vi "CLD 12 Sequencer State Machine.vi"() -> ()   [LabVIEW 2014]
doc: "CLD-Übung 12"
uses:
  CLD 12 Sequencer Enum.ctl
  CLD12 Timer Enum.ctl
  CLD 12 Data Cluster.ctl
panel:
  out "Aktuelle Zielzeit":dbl
  in  "Stopp-Schaltfläche":bool
  out "Verstrichene Zeit":dbl
  out "Schalter 3":bool
  out "Schalter 2":bool
  out "Schalter 1":bool
  in  "Start":bool
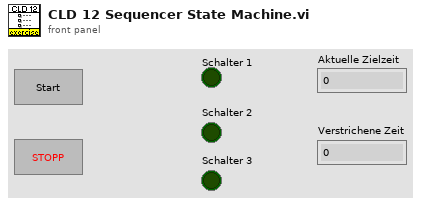
[diagram p1: front panel]
types:
  T1 = typedef "CLD 12 Sequencer Enum.ctl" = enum16{"Initialisieren", "SetTime", "RunState1", "Runstate2", "Ruhezustand", "Starten"}
  T2 = typedef "CLD12 Timer Enum.ctl" = enum16{"Timer starten", "Zeit lesen", "Anhalten", "Fortsetzen", "Timer zurücksetzen"}
  T3 = typedef "CLD 12 Data Cluster.ctl" = cluster{"Befehl":T1, "Zeitwert":dbl, "Boolesch":bool, "Boolesch 2":bool, "Boolesch 3":bool}
  T4 = cluster{"Status":bool, "Code":i32, "Quelle":string}
  T5 = cluster{string, "Zeitwert":dbl, "Boolesch":bool, "Boolesch 2":bool, "Boolesch 3":bool}
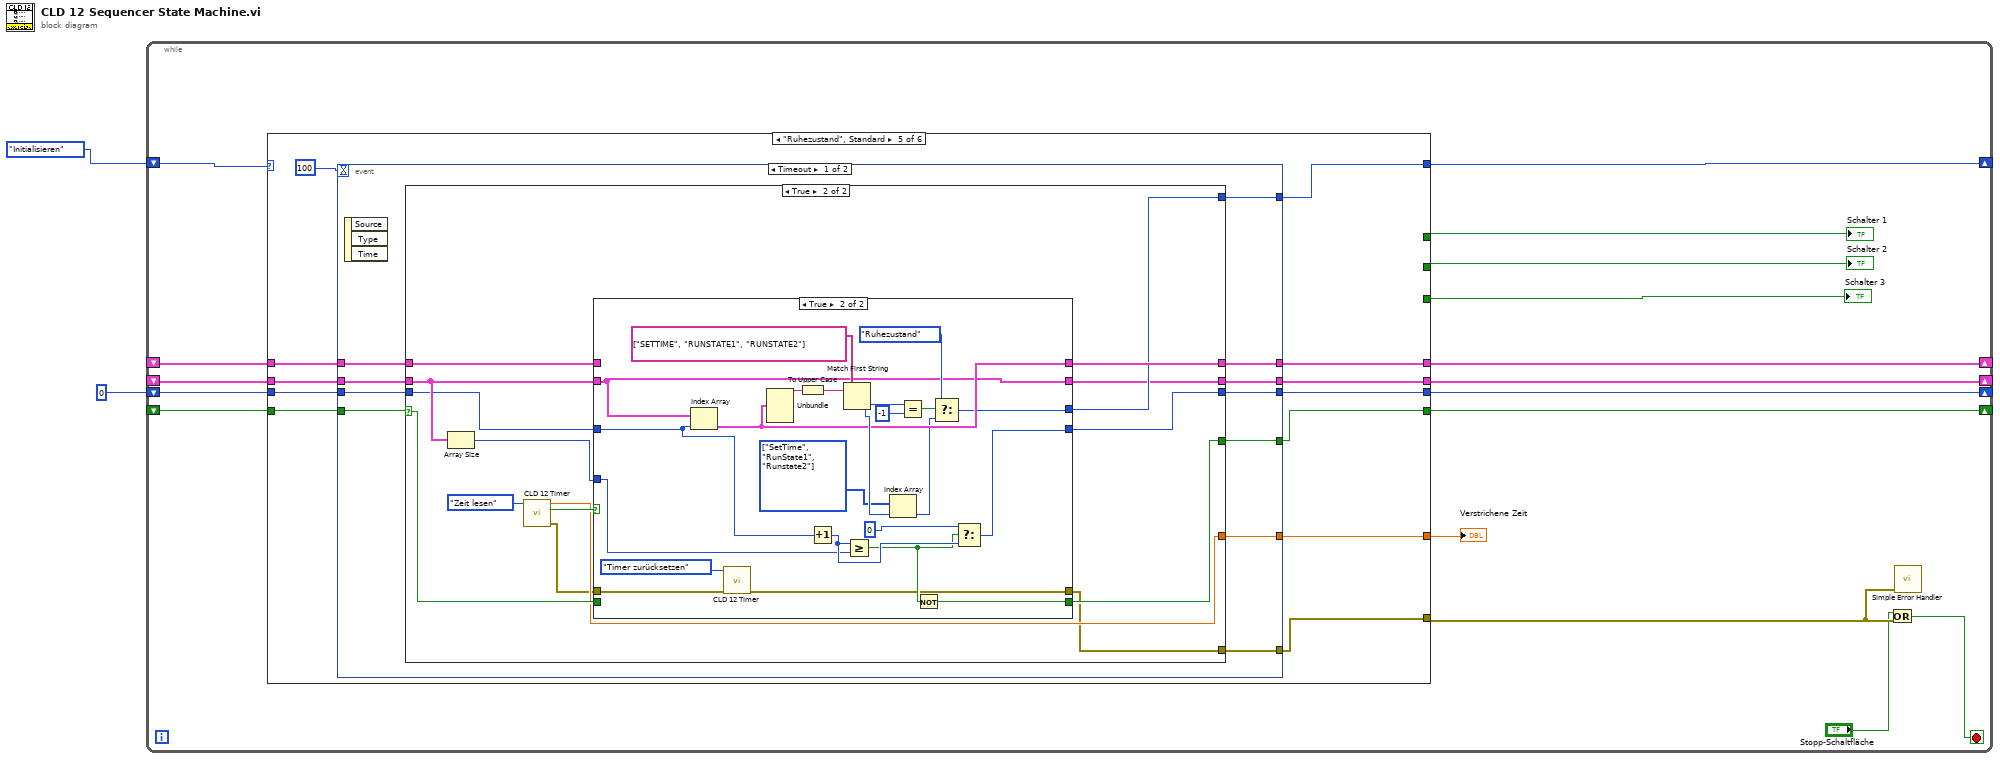
[diagram p0: block diagram]
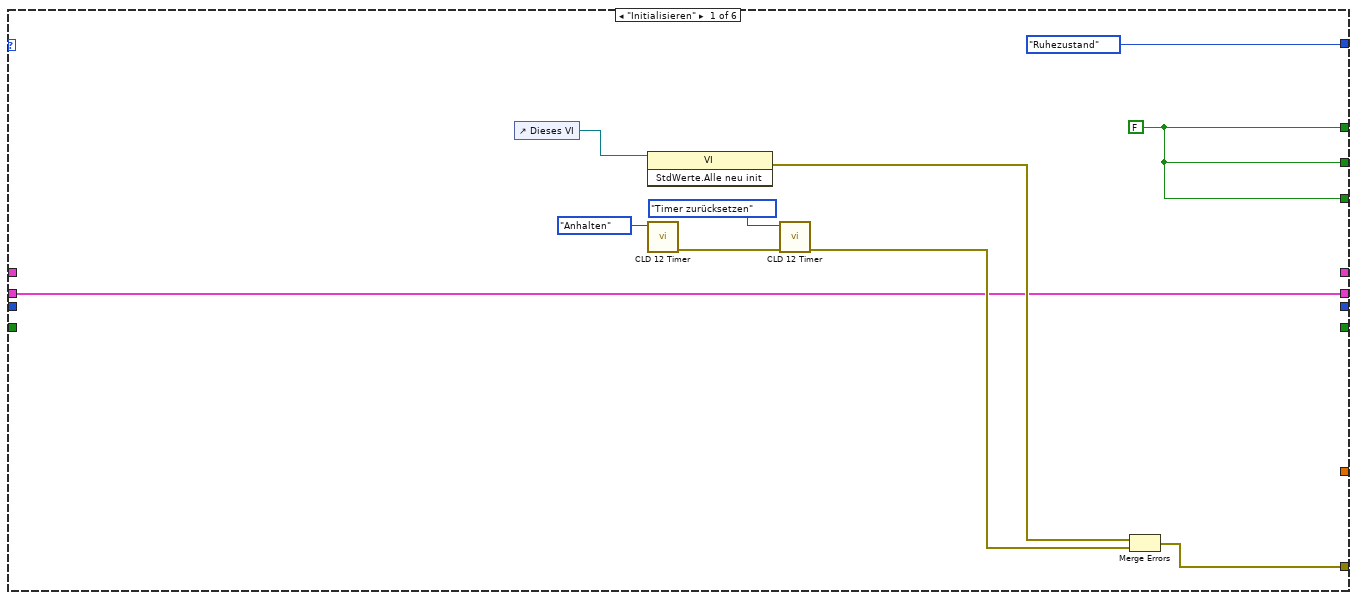
[diagram p2: hidden frame]
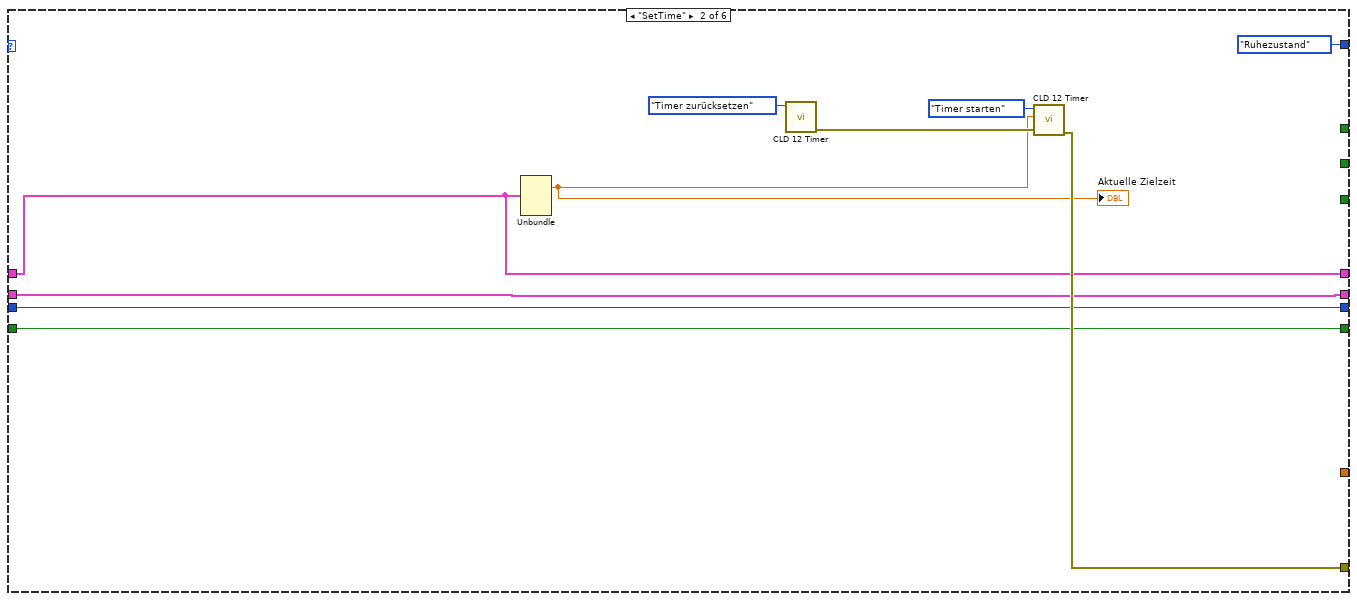
[diagram p3: hidden frame]
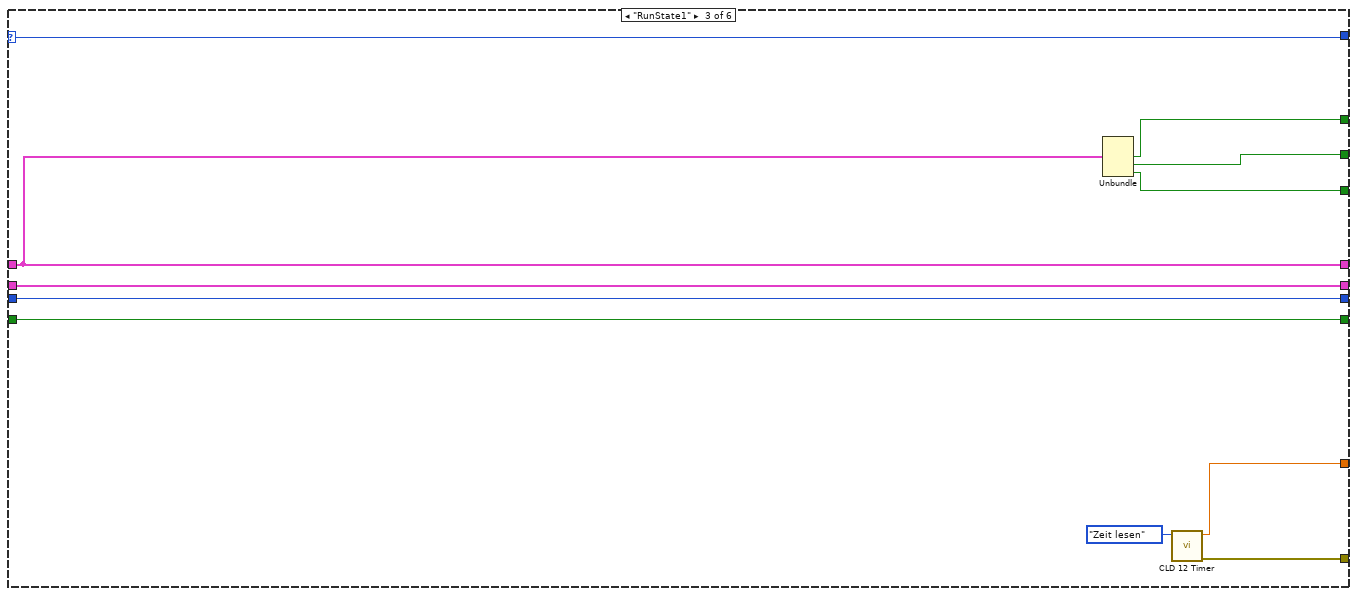
[diagram p4: hidden frame]
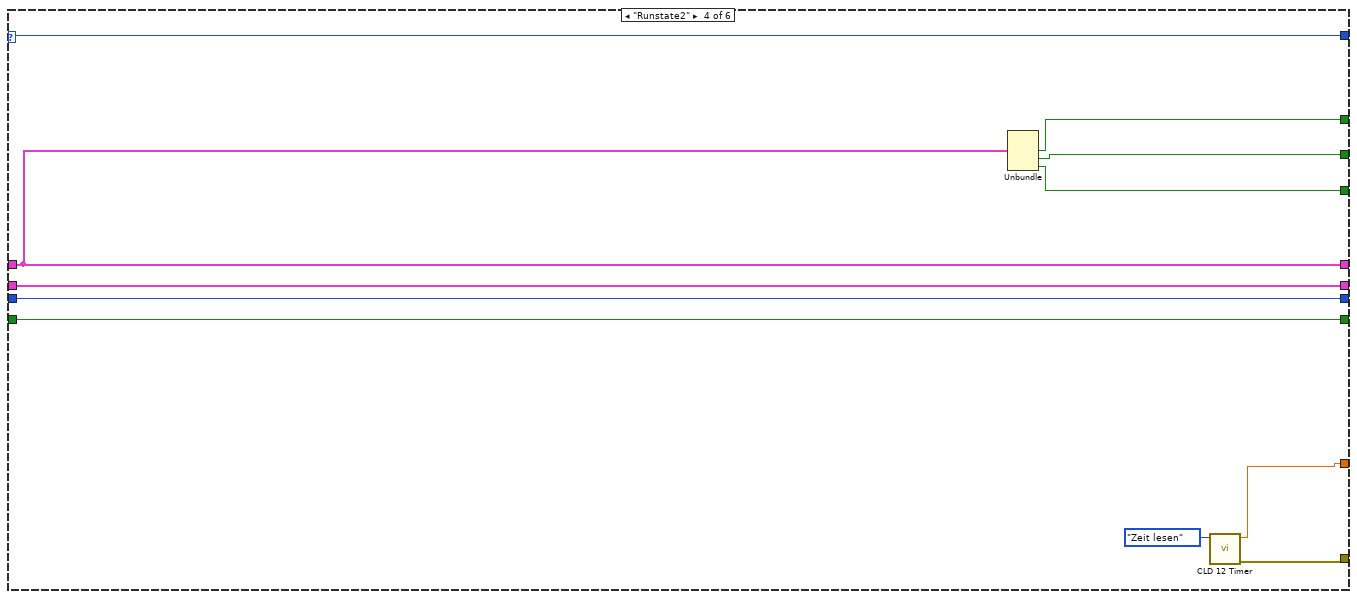
[diagram p5: hidden frame]
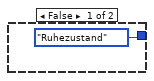
[diagram p6: hidden frame]
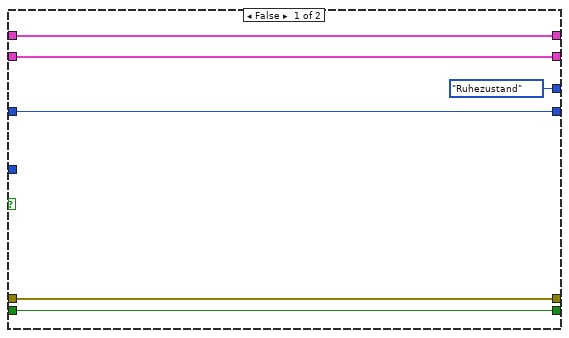
[diagram p7: hidden frame]
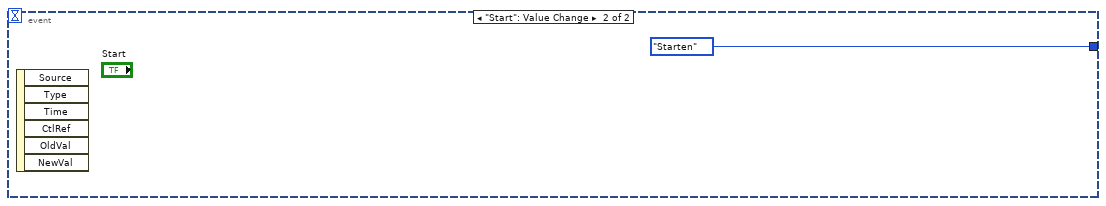
[diagram p8: hidden frame]
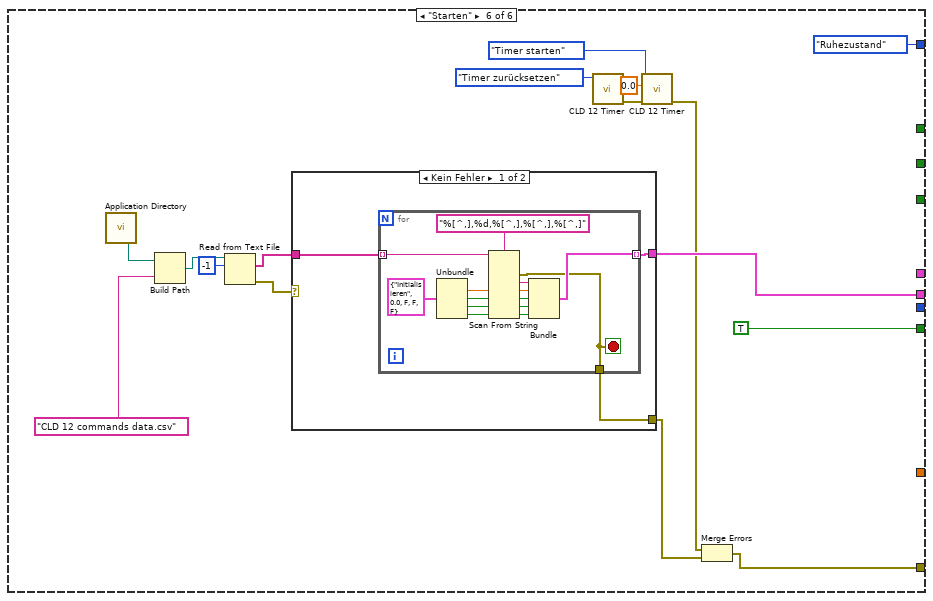
[diagram p9: hidden frame]
diagram:
  n1 = while {
    shift-right: [w10] -> _
    shift-left: CLD_12_Sequencer_Enum."Initialisieren" ("CLD 12 - Sequenzierelement") -> [w9]
    shift-right: [w14] -> _
    shift-left: _ -> [w8]
    shift-right: [w12] -> _
    shift-left: 0 -> [w5]
    shift-right: [w13] -> _
    shift-left: _ -> [w4]
    shift-right: [w6] -> _
    shift-left: _ -> [w7]
    stop <- w16 stop-if-true
    n2 = case shown="\"Ruhezustand\", Standard" w9 {
      selector: w9 -> [_ _ w50 w61 _ _]
      tunnel: [w28 _ w49 w60 _ _] -> w19
      tunnel: [w28 _ w48 w59 _ _] -> w18
      tunnel: [w28 _ w47 w58 _ _] -> w17
      tunnel: [w24 w38 w46 w56 w63 w136] -> w15
      tunnel: [w20 w34 w42 w54 w66 w137] -> w14
      tunnel: [_ w32 w40 w53 w65 TRUE] -> w13
      tunnel: [CLD_12_Sequencer_Enum."Ruhezustand" ("CLD 12 - Sequenzierelement") CLD_12_Sequencer_Enum."Ruhezustand" ("Befehl") w50 w61 w72 CLD_12_Sequencer_Enum."Ruhezustand" ("Befehl")] -> w10
      tunnel: [_ w33 w43 w51 w67 _] -> w12
      tunnel: w8 -> [w20 w34 w42 w54 w71 _]
      tunnel: w7 -> [_ w31 w41 w52 w69 _]
      tunnel: [_ w31 w41 w52 w70 _] -> w6
      tunnel: w5 -> [_ w33 w43 w51 w68 _]
      tunnel: w4 -> [_ w32 w40 w53 w64 _]
      tunnel: [_ _ w45 w55 w62 _] -> w3
      frame "Initialisieren" {
        w28 = FALSE
        n3 = control-ref of="Dieses VI"() -> (w29:refnum<vi>)
        n4 = invoke class="VI" method="StdWerte.Alle neu init"(reference=w29) -> (error out=w26:errorcluster)  [unwired: 2 in, 2 out]
        n5 = call "CLD 12 Timer.vi"("CLD 12 - Timer-Enum"=CLD12_Timer_Enum."Anhalten") -> ("Fehler (Ausgang)"=w25:T4)  [unwired: 8 in, 2 out]
        n6 = call "CLD 12 Timer.vi"("Fehler (Eingang)"=w25, "CLD 12 - Timer-Enum"=CLD12_Timer_Enum."Timer zurücksetzen") -> ("Fehler (Ausgang)"=w23:T4)  [unwired: 7 in, 2 out]
        n7 = Merge Errors(w26, w23) -> (w24:errorcluster)
      }
      frame "SetTime" {
        n8 = Unbundle(w31) -> ("Zeitwert"=w35:dbl)  [unwired: 4 out]
        "Aktuelle Zielzeit" <- w35
        n9 = call "CLD 12 Timer.vi"("CLD 12 - Timer-Enum"=CLD12_Timer_Enum."Timer zurücksetzen") -> ("Fehler (Ausgang)"=w37:T4)  [unwired: 8 in, 2 out]
        n10 = call "CLD 12 Timer.vi"("Fehler (Eingang)"=w37, "Zielzeit (s)"=w35, "CLD 12 - Timer-Enum"=CLD12_Timer_Enum."Timer starten") -> ("Fehler (Ausgang)"=w38:T4)  [unwired: 6 in, 2 out]
      }
      frame "RunState1" {
        n11 = Unbundle(w41) -> ("Boolesch"=w49:bool, "Boolesch 2"=w48:bool, "Boolesch 3"=w47:bool)  [unwired: 2 out]
        n12 = call "CLD 12 Timer.vi"("CLD 12 - Timer-Enum"=CLD12_Timer_Enum."Zeit lesen") -> ("Fehler (Ausgang)"=w46:T4, "Verstrichene Zeit (s,ms)"=w45:dbl)  [unwired: 8 in, 1 out]
      }
      frame "Runstate2" {
        n13 = Unbundle(w52) -> ("Boolesch"=w60:bool, "Boolesch 2"=w59:bool, "Boolesch 3"=w58:bool)  [unwired: 2 out]
        n14 = call "CLD 12 Timer.vi"("CLD 12 - Timer-Enum"=CLD12_Timer_Enum."Zeit lesen") -> ("Fehler (Ausgang)"=w56:T4, "Verstrichene Zeit (s,ms)"=w55:dbl)  [unwired: 8 in, 1 out]
      }
      frame "Ruhezustand", Default {
        n15 = event shown="[0] Timeout" {
          selector: _ -> [_ _]
          dyn-events: _ -> [_ _]
          timeout: 100 -> [_ _]
          tunnel: [w84 _] -> w70
          tunnel: [w83 CLD_12_Sequencer_Enum."Starten" ("Befehl")] -> w72
          tunnel: [w82 _] -> w67
          tunnel: [w80 _] -> w65
          tunnel: [w81 _] -> w63
          tunnel: w71 -> [w79 _]
          tunnel: w69 -> [w78 _]
          tunnel: w68 -> [w77 _]
          tunnel: [w76 _] -> w66
          tunnel: w64 -> [w75 _]
          tunnel: [w74 _] -> w62
          event Timeout {
            n16 = event-data() -> ()  [unwired: 1 in, 3 out]
            n17 = case shown="True" w75 {
              selector: w75 -> [_ w96]
              tunnel: [_ w94] -> w84
              tunnel: [CLD_12_Sequencer_Enum."Ruhezustand" ("Befehl") w93] -> w83
              tunnel: [_ w97] -> w82
              tunnel: [_ w86] -> w81
              tunnel: [_ w95] -> w80
              tunnel: w79 -> [_ w91]
              tunnel: w78 -> [_ w92]
              tunnel: w77 -> [_ w90]
              tunnel: [_ w89] -> w76
              tunnel: [_ w88] -> w74
              frame False {
              }
              frame True {
                n18 = Array Size(array=w91) -> (size(s)=w98:i32)
                n19 = call "CLD 12 Timer.vi"("CLD 12 - Timer-Enum"=CLD12_Timer_Enum."Zeit lesen") -> ("Fehler (Ausgang)"=w87:T4, "Ist Zeit verstrichen?"=w99:bool, "Verstrichene Zeit (s,ms)"=w88:dbl)  [unwired: 8 in]
                n20 = case shown="True" w99 {
                  tunnel: w98 -> [_ w126]
                  tunnel: [w105 w125] -> w97
                  tunnel: w96 -> [w106 _]
                  tunnel: [w106 w123] -> w95
                  tunnel: [w104 w114] -> w94
                  tunnel: [CLD_12_Sequencer_Enum."Ruhezustand" ("Befehl") w112] -> w93
                  tunnel: w91 -> [w103 w110]
                  tunnel: w92 -> [w104 _]
                  tunnel: w90 -> [w105 w111]
                  tunnel: [w103 w110] -> w89
                  tunnel: w87 -> [w101 w108]
                  tunnel: [w101 w107] -> w86
                  frame False {
                  }
                  frame True {
                    w118 = T1[] [enum."SetTime", enum."RunState1", enum."Runstate2"] items=["Initialisieren", "SetTime", "RunState1", "Runstate2", "Ruhezustand", "Starten"]
                    n21 = Index Array(array=w110, index=w111) -> (element=w114:T5)
                    n22 = call "CLD 12 Timer.vi"("Fehler (Eingang)"=w108, "CLD 12 - Timer-Enum"=CLD12_Timer_Enum."Timer zurücksetzen") -> ("Fehler (Ausgang)"=w107:T4)  [unwired: 7 in, 2 out]
                    n23 = Unbundle(w114) -> (w115:string)  [unwired: 4 out]
                    n24 = To Upper Case(1:w115) -> (0:w117:string)
                    n25 = Increment(x=w111) -> (x+1=w128:i32)
                    n26 = Match First String(2:string[] ["SETTIME", "RUNSTATE1", "RUNSTATE2"] ("String-Array"), 3:w117) -> (0:w119:i32)  [unwired: 1 out]
                    n27 = Greater Or Equal?(x=w128, y=w126) -> (x >= y?=w124:bool)
                    n28 = Index Array(array=w118, index=w119) -> (element=w113:T1)
                    n29 = Equal?(x=w119, y=-1) -> (x = y?=w121:bool)
                    n30 = Not(x=w124) -> (.not. x?=w123:bool)
                    n31 = Select(t=CLD_12_Sequencer_Enum."Ruhezustand", s=w121, f=w113) -> (s? t:f=w112:T1)
                    n32 = Select(t=0, s=w124, f=w128) -> (s? t:f=w125:i32)
                  }
                }
              }
            }
          }
          event "Start": Value Change {
            n33 = event-data() -> ()  [unwired: 1 in, 6 out]
          }
        }
      }
      frame "Starten" {
        n34 = call <vilib>:"Application Directory.vi"() -> ("Application Directory"=w142:path)
        n35 = Build Path(base path=w142, name or relative path="CLD 12 commands data.csv" ("Name oder relativer Pfad")) -> (appended path=w143:path)
        n36 = Read from Text File(file (use dialog)=w143, count=-1 ("Anzahl")) -> (text=w138:string[], error out=w139:errorcluster)  [unwired: 2 in, 2 out]
        n37 = case shown="Kein Fehler" w139 {
          selector: w139 -> [_ w163]
          tunnel: w138 -> [w148 _]
          tunnel: [w146 w163] -> w134
          tunnel: [w147 _] -> w137
          frame No Error {
            n38 = for {
              tunnel: w148 -> [w162] mode=indexing
              tunnel: [w150] -> w147 mode=indexing
              tunnel: [w149] -> w146
              stop <- w149 stop-if-true
              n39 = Unbundle(T3 {"Befehl"=enum."Initialisieren", "Zeitwert"=0.0, "Boolesch"=FALSE, "Boolesch 2"=FALSE, "Boolesch 3"=FALSE} ("CLD 12 - Daten-Cluster")) -> ("Zeitwert"=w159:dbl, "Boolesch"=w158:bool, "Boolesch 2"=w157:bool, "Boolesch 3"=w156:bool)  [unwired: 1 out]
              n40 = Scan From String(format string="%[^,],%d,%[^,],%[^,],%[^,]" ("Format-String"), input string=w162, default 2=w159, default 3=w158, default 4=w157, default 5=w156) -> (error out=w149:errorcluster, output 1=w155:string, output 2=w154:dbl, output 3=w153:bool, output 4=w152:bool, output 5=w151:bool)  [unwired: 3 in, 2 out]
              n41 = Bundle(w155, "Zeitwert"=w154, "Boolesch"=w153, "Boolesch 2"=w152, "Boolesch 3"=w151) -> (w150:T5)  [unwired: 1 in]
            }
          }
          frame Error {
          }
        }
        n42 = call "CLD 12 Timer.vi"("CLD 12 - Timer-Enum"=CLD12_Timer_Enum."Timer zurücksetzen") -> ("Fehler (Ausgang)"=w135:T4)  [unwired: 8 in, 2 out]
        n43 = call "CLD 12 Timer.vi"("Fehler (Eingang)"=w135, "Zielzeit (s)"=0.0, "CLD 12 - Timer-Enum"=CLD12_Timer_Enum."Timer starten") -> ("Fehler (Ausgang)"=w132:T4)  [unwired: 6 in, 2 out]
        n44 = Merge Errors(w132, w134) -> (w136:errorcluster)
      }
    }
    "Schalter 1" <- w19
    "Schalter 2" <- w18
    "Schalter 3" <- w17
    "Verstrichene Zeit" <- w3
    n45 = Or(x="Stopp-Schaltfläche", y=w15) -> (x .or. y?=w16:bool)
    n46 = call <vilib>:"Simple Error Handler.vi"("error in (no error)"=w15) -> ()  [unwired: 4 in, 5 out]
  }
